vi "Recursion Solution.vi"() -> ()   [LabVIEW 2014]
uses:
  ctl/Coin data--cluster.ctl
panel:
  in  "Update display?":bool
  out "Max Quantities":i32[](array[numeric])
  out "Solutions (Quantity)":i32[][](array[numeric])
  out "No. solutions":i32
  out "Values (£)":i32[](array[numeric])
  out "Time taken (s)":dbl
  # "Beer Money - Recursion Solution"
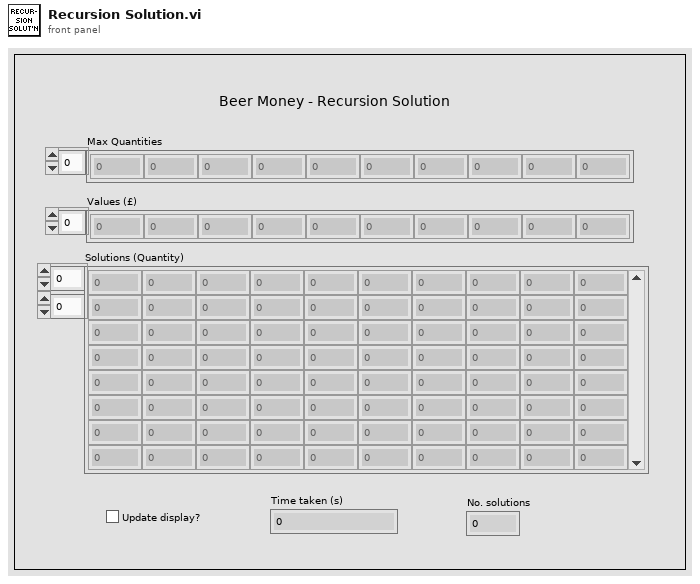
[diagram p1: front panel]
types:
  T1 = typedef "Coin data--cluster.ctl" = cluster{"Coin/note":i32, "Quantity":i32}
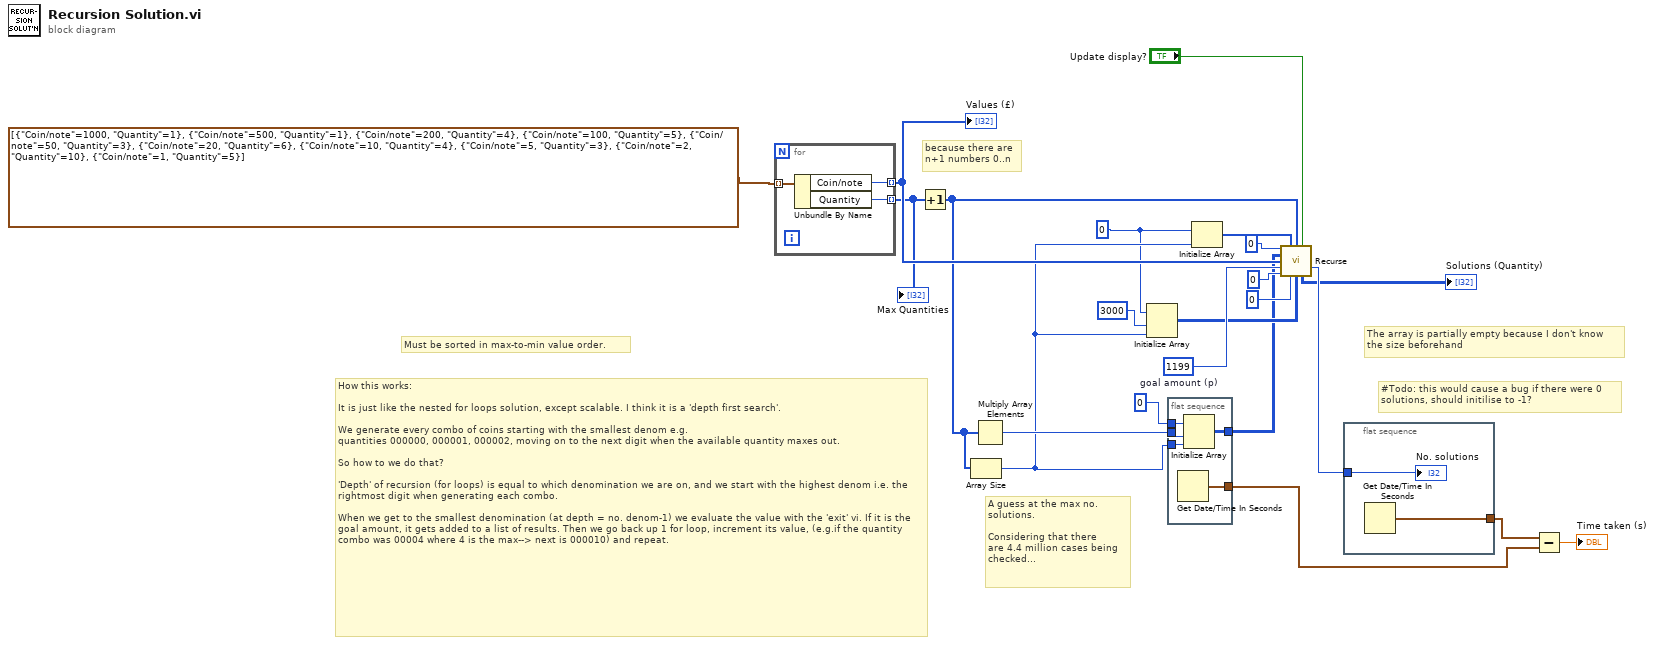
[diagram p0: block diagram]
diagram:
  w10 = 1199  # goal amount (p)
  w11 = 0
  # "How this works:\n\nIt is just like the nested for loops solution, except scalable. I think it is a 'depth first search'.\n\nWe generate every combo of coins starting with the smallest denom e.g.\nquantities 000000, 000001, 000002, moving on to the next digit when the available quantity maxes out.\n\nSo how to we do that?\n\n'Depth' of recursion (for loops) is equal to which denomination we are on, and we start with the highest denom i.e. the rightmost digit when generating each combo.\n\nWhen we get to the smallest denomination (at depth = no. denom-1) we evaluate the value with the 'exit' vi. If it is the goal amount, it gets added to a list of results. Then we go back up 1 for loop, increment its value, (e.g.if the quantity combo was 00004 where 4 is the max--> next is 000010) and repeat."
  # "A guess at the max no.\nsolutions.\n\nConsidering that there \nare 4.4 million cases being \nchecked..."
  # "#Todo: this would cause a bug if there were 0\nsolutions, should initilise to -1?"
  # "Must be sorted in max-to-min value order."
  # "The array is partially empty because I don't know\nthe size beforehand"
  # "because there are \nn+1 numbers 0..n"
  n1 = for {
    tunnel: T1[] [{"Coin/note"=1000, "Quantity"=1}, {"Coin/note"=500, "Quantity"=1}, {"Coin/note"=200, "Quantity"=4}, {"Coin/note"=100, "Quantity"=5}, {"Coin/note"=50, "Quantity"=3}, {"Coin/note"=20, "Quantity"=6}, {"Coin/note"=10, "Quantity"=4}, {"Coin/note"=5, "Quantity"=3}, {"Coin/note"=2, "Quantity"=10}, {"Coin/note"=1, "Quantity"=5}] -> [w25] mode=indexing
    tunnel: [w24] -> w18 mode=indexing
    tunnel: [w23] -> w2 mode=indexing
    n2 = Unbundle By Name(w25) -> ("Coin/note"=w24:i32, "Quantity"=w23:i32)
  }
  "Values (£)" <- w18
  "Max Quantities" <- w2
  n3 = Increment(x=w2) -> (x+1=w15:i32[])
  n4 = Array Size(array=w15) -> (size(s)=w16:i32)
  n5 = Multiply Array Elements(1:w15) -> (0:w22:i32)
  n6 = Initialize Array(w11, 3000 ("dimension size"), w16) -> (w8:i32[][])
  n7 = flat-sequence {
    tunnel: w22 -> [w30]
    tunnel: [w29] -> w21
    tunnel: w16 -> [w28]
    tunnel: 0 ("dimension size") -> [w27]
    tunnel: [w26] -> w5
    frame #0 {
      n8 = Get Date/Time In Seconds() -> (seconds since 1Jan1904=w29:timestamp)
      n9 = Initialize Array(w27, w30, w28) -> (w26:i32[][])
    }
  }
  n10 = Initialize Array(w11, w16) -> (w14:i32[])
  n11 = call "Recurse.vi"("Combo index in"=0 ("combo index in"), "Iterations array in"=w14, "Quantities"=w15, "Update display?"="Update display?", "Combos in"=w5, "Values"=w18, "Goal amount"=w10, "Depth"=0, "Result index in"=0 ("result index in"), "Results in"=w8) -> ("Result index out"=w17:i32, "Results out"=→"Solutions (Quantity)":i32[][])  [unwired: 1 in, 3 out]
  n12 = flat-sequence {
    tunnel: [w32] -> w20
    tunnel: w17 -> [w31]
    frame #0 {
      n13 = Get Date/Time In Seconds() -> (seconds since 1Jan1904=w32:timestamp)
      "No. solutions" <- w31
    }
  }
  n14 = Subtract(x=w20, y=w21) -> (x-y=→"Time taken (s)":dbl)
